vi "qRMC.vi"(0 "System no.":i32=1 min=1 max=4 step=1, 5 "error in":errorcluster) -> (14 "Running macros":string, 19 "error out":errorcluster)   [LabVIEW 2026]
doc: "List macros currently running.\n\nC-887, F-206, M-8X0: Only for GCS syntax version = GCS 2.0 or higher (check with CSV?.vi. If CSV?.vi is not supported, syntax version is GCS 1.0)."
panel:
  # "List macros currently running"
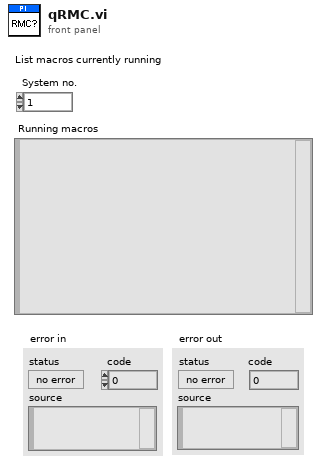
[diagram p1: front panel]
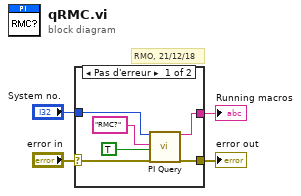
[diagram p0: block diagram]
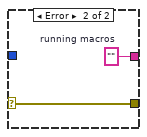
[diagram p2: hidden frame]
diagram:
  # "RMO, 21/12/18"
  n1 = case shown="Pas d'erreur" "error in" {
    selector: "error in" -> [w7 w12]
    tunnel: [w5 w11] -> w4
    tunnel: [w6 w12] -> w3
    tunnel: "System no." -> [w8 _]
    frame No Error {
      n2 = call "PI Query.vi"("System no."=w8, "String to send"="RMC?" ("String to Send"), "Attach termination char.?"=TRUE ("Attach Linefeed?"), "error in"=w7) -> ("String read"=w5:string, "error out"=w6:errorcluster)  [unwired: 3 in, 11 out]
    }
    frame Error {
      w11 = ""  # running macros
    }
  }
  "Running macros" <- w4
  "error out" <- w3
